vi "Pattern Example.vi"() -> ()   [LabVIEW 2014]
uses:
  <vilib>/Platform/TimedLoop/XDataNode/timing_clust.ctl
  <vilib>/Platform/TimedLoop/XDataNode/nitl_modes.ctl
  <vilib>/Platform/TimedLoop/XDataNode/wakeup.ctl
  <vilib>/rvi/Emulation/niFpgaSctlEmulationGetInTimedLoop.vi
  <vilib>/rvi/Emulation/niFpgaEmulationReportErrorSimple.vi
  <vilib>/rvi/Emulation/niFpgaGetClockAttributes.vi
  <vilib>/rvi/Emulation/niFpgaCriticalErrorInLSC.vi
  <vilib>/rvi/eio/common/nirviEmuTemplateMethod_errors.vi
  <vilib>/rvi/Emulation/niFpgaEmulationIsFPGAContextNoSignature.vi
  <vilib>/rvi/errors/niFpgaSetErrorForExecOnDevCompSimple.vi
  <vilib>/rvi/eio/common/nirviEmuReportErrorAndStop.vi
  <vilib>/rvi/DataTransferAndStorage/Container/Common/niFpgaContainerGetUniqueNameForEmu.vi
  <vilib>/rvi/FIFO/Fifo_Resource/nirvififoEmulationSetSize.vi
  <vilib>/rvi/FIFO/Fifo_Resource/nirviFifoEmulationQueueMgr.vi
  <instcachedir>/0/nirviFifoEmulationQueueMgr_E5CAEC123FF24DC58D834DCA3CDAA9B5.lvgen/nirviFifoEmulationQueueMgr_E5CAEC123FF24DC58D834DCA3CDAA9B5_006.vi
  <vilib>/rvi/FIFO/Fifo_Resource/nirvififoEmulationDetermineInputValidOut.vi
  <vilib>/rvi/FIFO/Fifo_Resource/nirvififoEmulationCreateLock.vi
  <vilib>/rvi/Emulation/niFpgaProcessEmulError.vi
  <vilib>/rvi/FIFO/Fifo_Resource/nirvififoEmulationObtainLock.vi
  <vilib>/rvi/FIFO/Fifo_Resource/nirvififoEmulationReleaseLock.vi
  <vilib>/rvi/occurrence/nirviWaitOnOccurrenceBase.vi
  <vilib>/rvi/errors/nirviReportUnexpectedCaseInternalError.vi
  <vilib>/rvi/errors/nirviReportUnexpectedCaseInternalError (U32).vi
  <vilib>/rvi/interface/RandomDataEmulation/niFpgaRandomDataHandleErrors.vi
  <vilib>/Platform/TimedLoop/XDataNode/XDataNode.xnode
  <vilib>/eio/EIONode/EIONode.xnode
  <vilib>/rvi/DataTransferAndStorage/Container/XNode/niFpgaContainer.xnode
  <vilib>/rvi/FIFO/Fifo_Resource/nirvififoEmulationWrite.vi
  <vilib>/rvi/FIFO/Fifo_Resource/nirvififoEmulationRead.vi
  <vilib>/rvi/interface/RandomDataEmulation/nirviRandomDataFpgaReadWriteTemplate.vi
  <vilib>/Platform/TimedLoop/XDataNode/XDNodeRunTimeDep.lvlib
panel:
  out "Numeric":i32
  in  "clear":bool
  out "Overflow":bool
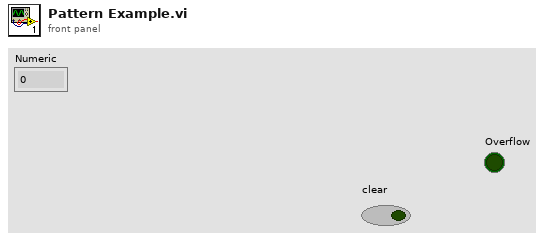
[diagram p1: front panel]
types:
  T1 = typedef "XDNodeRunTimeDep.lvlib/timing_clust.ctl" = cluster{"Expected End [f-1]":u64, "Actual End [f-1]":u64, "Finished Late? [f-1]":bool, "Expected End [i-1]":u64, "Actual End [i-1]":u64, "Finished Late? [i-1]":bool, "Expected Start [i]":u64, "Actual Start [i]":u64, "Expected Start [f]":u64, "Actual Start [f]":u64, "Source Name":string, "Structure Name":string, "Period":i64, "Deadline":i64, "Offset":i64, "Start":i64, "Priority":i32, "Timeout":i32, "Mode":T2, "Wakeup Reason":T3, "Error":errorcluster, "Source Type":string, "Secondary Source Type":string, "Global End Time":u64, "Global Start Time":u64, "Frame Duration":u64, "Iteration Duration":u64, "Assigned CPU":i32, "I/O Scan Engine Mode":u32}
  T2 = typedef "XDNodeRunTimeDep.lvlib/nitl_modes.ctl" = enum32{"No Change", "Process missed periods, maintain original phase", "Discard missed periods, maintain original phase", "Process missed periods, ignore original phase", "Discard missed periods, ignore original phase"}
  T3 = typedef "XDNodeRunTimeDep.lvlib/wakeup.ctl" = enum32{"Normal", "Aborted", "Asynchronous wakeup", "Timing source error", "Timed loop error", "Timeout"}
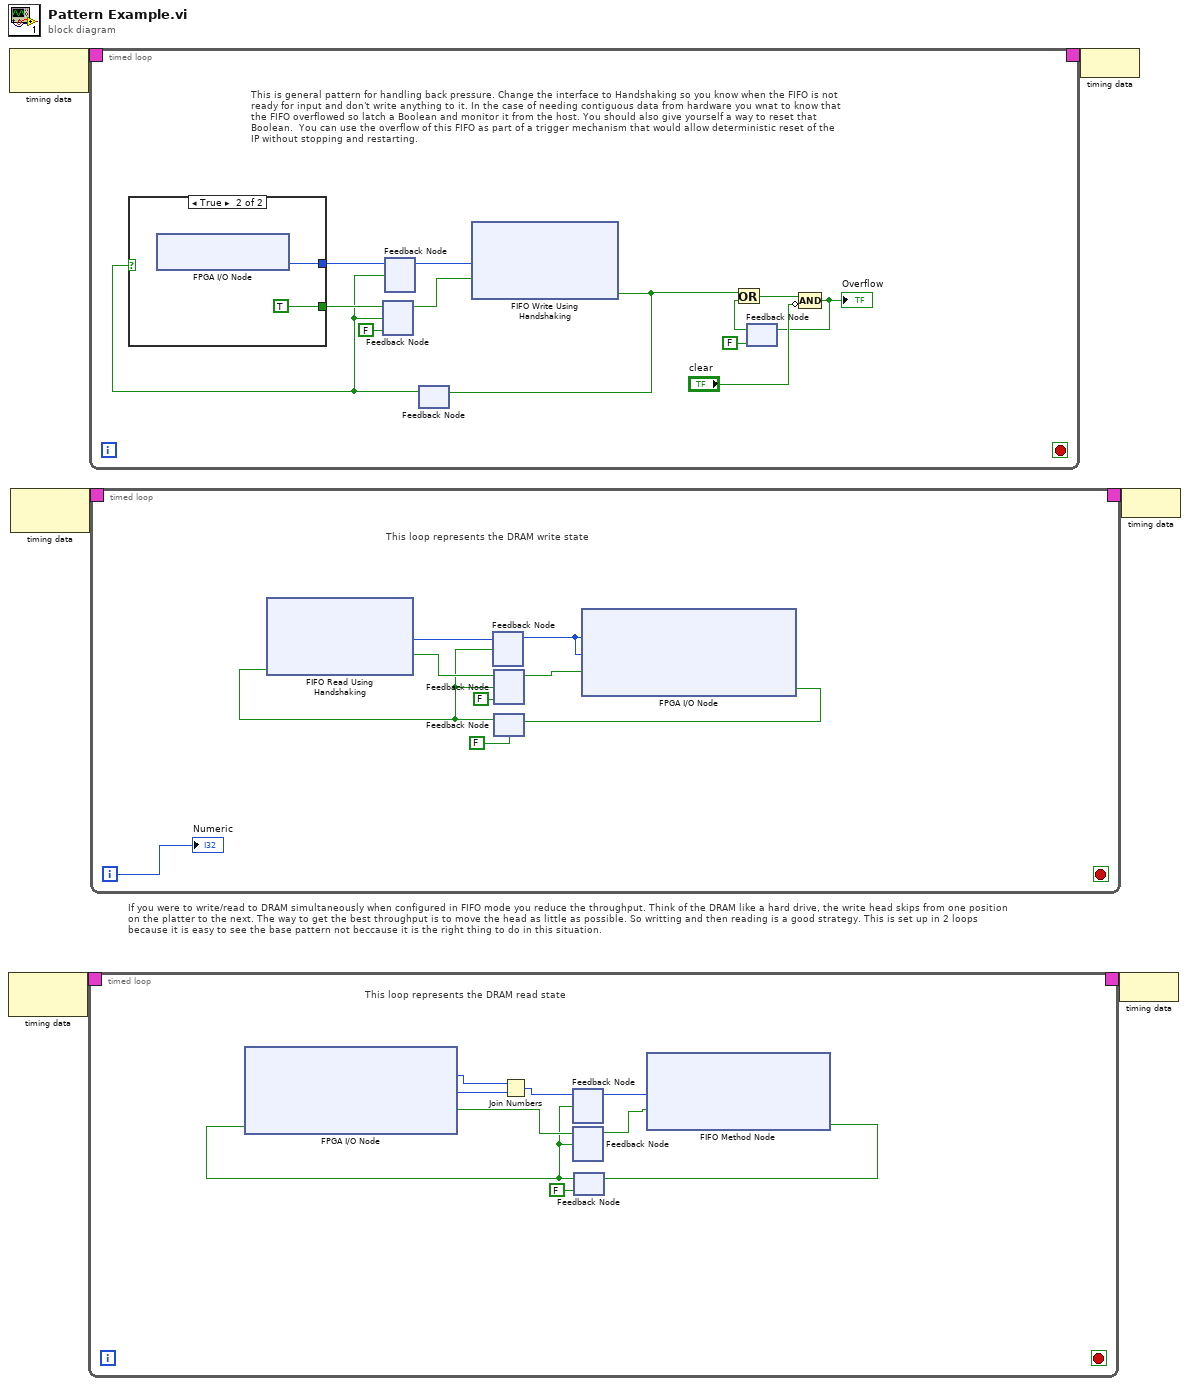
[diagram p0: block diagram]
diagram:
  # "If you were to write/read to DRAM simultaneously when configured in FIFO mode you reduce the throughput. Think of the DRAM like a hard drive, the write head skips from one position on the platter to the next. The way to get the best throughput is to move the head as little as possible. So writting and then reading is a good strategy. This is set up in 2 loops because it is easy to see the base pattern not beccause it is the right thing to do in this situation."
  n1 = node-c288() -> (w2:T1)  [unwired: 1 in]
  n2 = node-c288() -> (w6:T1)  [unwired: 1 in]
  n3 = node-c288() -> (w4:T1)  [unwired: 1 in]
  n4 = timed-loop {
    timing: w2 -> [_]
    timing-out: [_] -> w1
    stop <- _ stop-if-true
    # "This loop represents the DRAM read state"
    n5 = feedback #1() -> (w8:u64)  [unwired: 1 in]
    n6 = feedback #2() -> (w9:bool)  [unwired: 1 in]
    n7 = feedback #3(FALSE ("Ready for Input")) -> (w7:bool)
    n8 = xnode "FPGA I/O Node"("DRAM Bank 0\\Read"=w7) -> ("DRAM Bank 0\\Read_Data_Upper"=w13:u32, "DRAM Bank 0\\Read_Data_Lower"=w12:u32, "DRAM Bank 0\\Data_Available"=w10:bool)  [unwired: 4 in, 4 out]
    n9 = Join Numbers(hi=w13, lo=w12) -> ((hi.lo)=w11:u64)
    n10 = feedback-in #1(w11, w7) -> ()
    n11 = feedback-in #2(w10, w7) -> ()
    n12 = xnode ("FIFO Method Node")("Element"=w8, "Input Valid"=w9) -> ("Ready for Input"=w15:bool)  [unwired: 1 in, 1 out]
    n13 = feedback-in #3(w15) -> ()
  }
  n14 = timed-loop {
    timing: w6 -> [_]
    timing-out: [_] -> w5
    stop <- _ stop-if-true
    # "This is general pattern for handling back pressure. Change the interface to Handshaking so you know when the FIFO is not ready for input and don't write anything to it. In the case of needing contiguous data from hardware you wnat to know that the FIFO overflowed so latch a Boolean and monitor it from the host. You should also give yourself a way to reset that Boolean.  You can use the overflow of this FIFO as part of a trigger mechanism that would allow deterministic reset of the IP without stopping and restarting."
    n15 = feedback #4(FALSE) -> (w24:bool)
    n16 = feedback #5() -> (w28:i16)  [unwired: 1 in]
    n17 = feedback #6() -> (w26:bool)  [unwired: 1 in]
    n18 = case shown="True" w26 {
      tunnel: [_ w31] -> w29
      tunnel: [_ TRUE] -> w27
      frame False {
      }
      frame True {
        n19 = xnode "FPGA I/O Node"() -> ("IO Module\\AI A0"=w31:i16)  [unwired: 1 in, 1 out]
      }
    }
    n20 = feedback-in #4(w27, w26) -> ()
    n21 = feedback-in #5(w29, w26) -> ()
    n22 = xnode "FIFO Write Using Handshaking"("Element"=w28, "Input Valid"=w24) -> ("Ready for Input"=w18:bool)  [unwired: 1 in, 1 out]
    n23 = feedback-in #6(w18) -> ()
    n24 = feedback #7(FALSE) -> (w19:bool)
    n25 = Or(x=w18, y=w19) -> (x .or. y?=w22:bool)
    n26 = Compound Arithmetic op=AND(w22, invert "clear") -> (w21:bool)
    "Overflow" <- w21
    n27 = feedback-in #7(w21) -> ()
  }
  n28 = timed-loop {
    timing: w4 -> [_]
    timing-out: [_] -> w3
    i -> [w34]
    stop <- _ stop-if-true
    # "This loop represents the DRAM write state"
    n29 = feedback #8() -> (w41:u32)  [unwired: 1 in]
    n30 = feedback #9(FALSE ("Output Valid")) -> (w38:bool)
    n31 = feedback #10(FALSE ("DRAM Bank 0\\Full")) -> (w35:bool)
    n32 = xnode "FIFO Read Using Handshaking"("Ready for Output"=w35) -> ("Element"=w42:u32, "Output Valid"=w40:bool)  [unwired: 1 in, 1 out]
    n33 = feedback-in #8(w42, w35) -> ()
    n34 = feedback-in #9(w40, w35) -> ()
    n35 = xnode "FPGA I/O Node"("DRAM Bank 0\\Write_Data_Upper"=w41, "DRAM Bank 0\\Write_Data_Lower"=w41, "DRAM Bank 0\\Write"=w38) -> ("DRAM Bank 0\\Full"=w37:bool)  [unwired: 4 in, 4 out]
    n36 = feedback-in #10(w37) -> ()
    "Numeric" <- w34
  }
  n37 = node-c288(w5) -> ()
  n38 = node-c288(w1) -> ()
  n39 = node-c288(w3) -> ()
